vi "Create Response.vi"(8 "error in (no error)":errorcluster, 10 "result":variant, 11 "Response":refnum<class "Response.lvclass">) -> (0 "error out":errorcluster, 2 "JSON Response":string, 3 "Response out":refnum<class "Response.lvclass">)   [LabVIEW 2019, in "Response.lvclass"]
uses:
  Response.lvclass
  Response.lvclass/Response.ctl
  typedefs/Error Object--Cluster.ctl
  lv-venv/lv.lib/user.lib/_OpenG.lib/error/error.llb/Filter Error Codes (Array)__ogtk.vi
  lv-venv/lv.lib/vi.lib/addons/_JKI.lib/Serialization/JSON/JKI JSON Serialization.lvlib
  JSON-RPC.lvclass
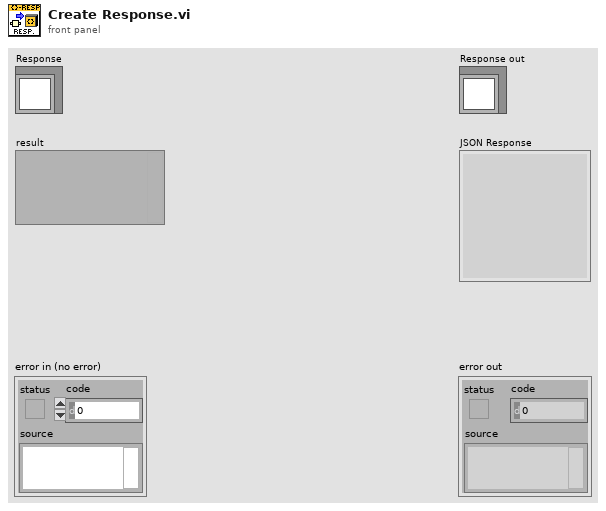
[diagram p1: front panel]
types:
  T1 = typedef "JSON-RPC.lvclass/Error Object--Cluster.ctl" = cluster{"code":i32, "message":string, "data":variant}
  T2 = cluster{"jsonrpc":string, "result":variant, "id":string}
  T3 = cluster{"jsonrpc":string, "Error":T1, "id":string}
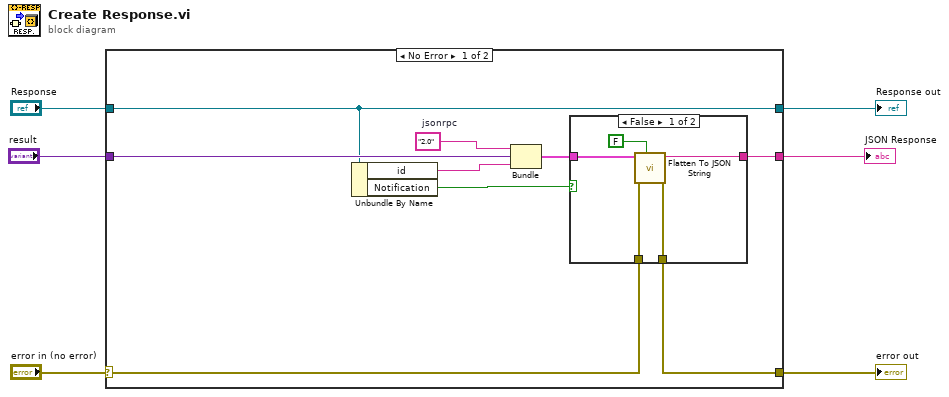
[diagram p0: block diagram]
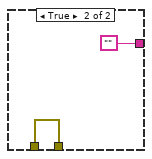
[diagram p2: hidden frame]
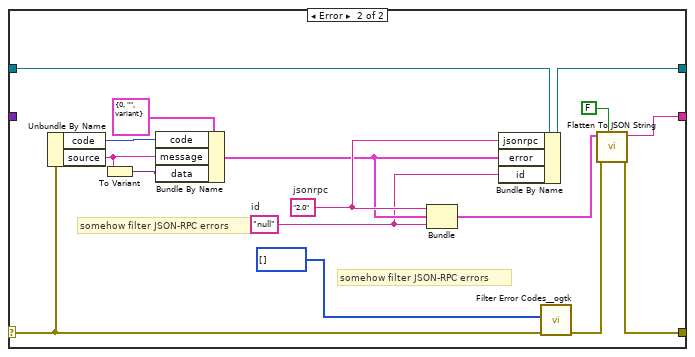
[diagram p3: hidden frame]
diagram:
  n1 = case shown="No Error" "error in (no error)" {
    selector: "error in (no error)" -> [w13 w35]
    tunnel: [w12 w25] -> w2
    tunnel: [w9 w33] -> w5
    tunnel: "Response" -> [w9 w34]
    tunnel: "result" -> [w11 _]
    tunnel: [w14 w24] -> w1
    frame No Error {
      w10 = "2.0"  # jsonrpc
      n2 = Unbundle By Name(w9) -> ("id"=w8:string, "Notification"=w7:bool)
      n3 = Bundle("jsonrpc"=w10, "result"=w11, "id"=w8) -> (w15:T2)  [unwired: 1 in]
      n4 = case shown="False" w7 {
        tunnel: w15 -> [w20 _]
        tunnel: [w18 ""] -> w14
        tunnel: w13 -> [w17 w22]
        tunnel: [w16 w22] -> w12
        frame False {
          n5 = call "Flatten To JSON String.vi"("Multiline (T)"=FALSE, "error in (no error)"=w17, "Variant"=w20) -> ("error out"=w16:errorcluster, "JSON String"=w18:string)  [unwired: 7 in]
        }
        frame True {
        }
      }
    }
    frame Error {
      w32 = "2.0"  # jsonrpc
      w30 = "null"  # id
      # "somehow filter JSON-RPC errors"
      # "somehow filter JSON-RPC errors"
      n6 = Unbundle By Name(w35) -> ("code"=w36:i32, "source"=w38:string)
      n7 = To Variant(anything=w38) -> (Variant=w37:variant)
      n8 = Bundle By Name(cluster=T1 {"code"=0, "message"="", "data"=variant} ("Error"), "code"=w36, "message"=w38, "data"=w37) -> (w31:T1)
      n9 = Bundle("jsonrpc"=w32, "Error"=w31, "id"=w30) -> (w27:T3)  [unwired: 1 in]
      n10 = Bundle By Name(cluster=w34, "jsonrpc"=w32, "error"=w31, "id"=w30) -> (w33:refnum<class "Response.lvclass">)
      n11 = call-poly "Filter Error Codes__ogtk.vi"("Error In"=w35, "Error Codes to Filter"=i32[] []) -> ("Error Out"=w26:errorcluster)  [unwired: 7 in, 2 out]
      n12 = call "Flatten To JSON String.vi"("Multiline (T)"=FALSE, "error in (no error)"=w26, "Variant"=w27) -> ("error out"=w25:errorcluster, "JSON String"=w24:string)  [unwired: 7 in]
    }
  }
  "error out" <- w2
  "Response out" <- w5
  "JSON Response" <- w1
